vi "Alarm-102.vi"() -> ()   [LabVIEW 2009]
panel:
  out "³Ñ¤UªººÎ¯v®É¶¡":string
  in  "MINUTE":i32
  in  "HOUR":i32
  in  "stop":bool
  out "TIME":T1
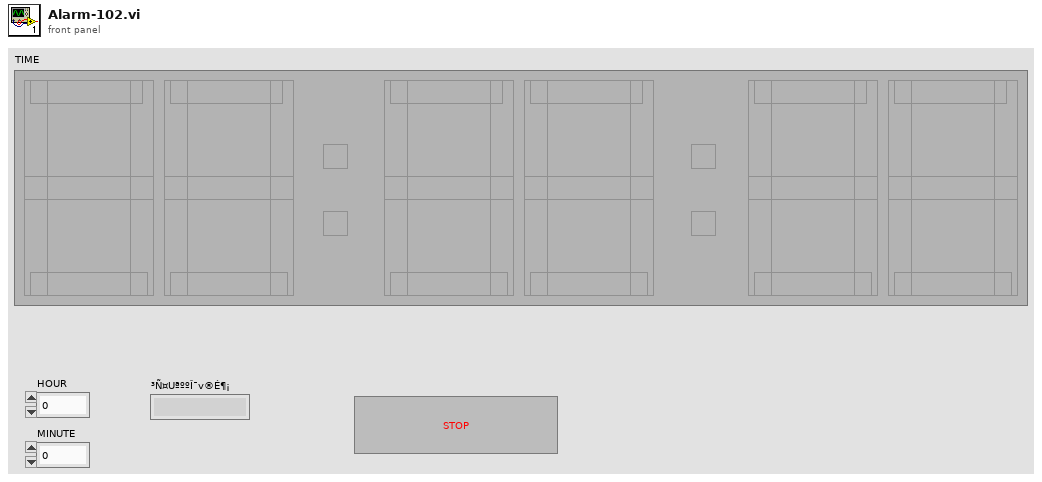
[diagram p1: front panel]
types:
  T1 = cluster{"Cluster":cluster{"Boolean 6":bool, "Boolean":bool, "Boolean 2":bool, "Boolean 7":bool, "Boolean 3":bool, "Boolean 4":bool, "Boolean 5":bool}, "Cluster 2":cluster{"Boolean 6":bool, "Boolean":bool, "Boolean 2":bool, "Boolean 7":bool, "Boolean 3":bool, "Boolean 4":bool, "Boolean 5":bool}, "Cluster 3":cluster{"Boolean 6":bool, "Boolean":bool, "Boolean 2":bool, "Boolean 7":bool, "Boolean 3":bool, "Boolean 4":bool, "Boolean 5":bool}, "Cluster 4":cluster{"Boolean 6":bool, "Boolean":bool, "Boolean 2":bool, "Boolean 7":bool, "Boolean 3":bool, "Boolean 4":bool, "Boolean 5":bool}, "Cluster 5":cluster{"Boolean 6":bool, "Boolean":bool, "Boolean 2":bool, "Boolean 7":bool, "Boolean 3":bool, "Boolean 4":bool, "Boolean 5":bool}, "Cluster 6":cluster{"Boolean 6":bool, "Boolean":bool, "Boolean 2":bool, "Boolean 7":bool, "Boolean 3":bool, "Boolean 4":bool, "Boolean 5":bool}, "sec1":bool, "sec2":bool, "sec2 2":bool, "sec1 2":bool}
  T2 = cluster{"Boolean 6":bool, "Boolean":bool, "Boolean 2":bool, "Boolean 7":bool, "Boolean 3":bool, "Boolean 4":bool, "Boolean 5":bool}[]
  T3 = typedef "LVDateTimeRec.ctl" = cluster{"fractional second":dbl, "second":i32, "minute":i32, "hour":i32, "day of month":i32, "month":i32, "year":i32, "day of week":i32, "day of year":i32, "DST":i32}
  T4 = cluster{"Boolean 6":bool, "Boolean":bool, "Boolean 2":bool, "Boolean 7":bool, "Boolean 3":bool, "Boolean 4":bool, "Boolean 5":bool}
  T5 = cluster{"second":i32, "minute":i32, "hour":i32, "day of month":i32, "month":i32, "year":i32, "day of week":i32, "day of year":i32, "is DST":i32}
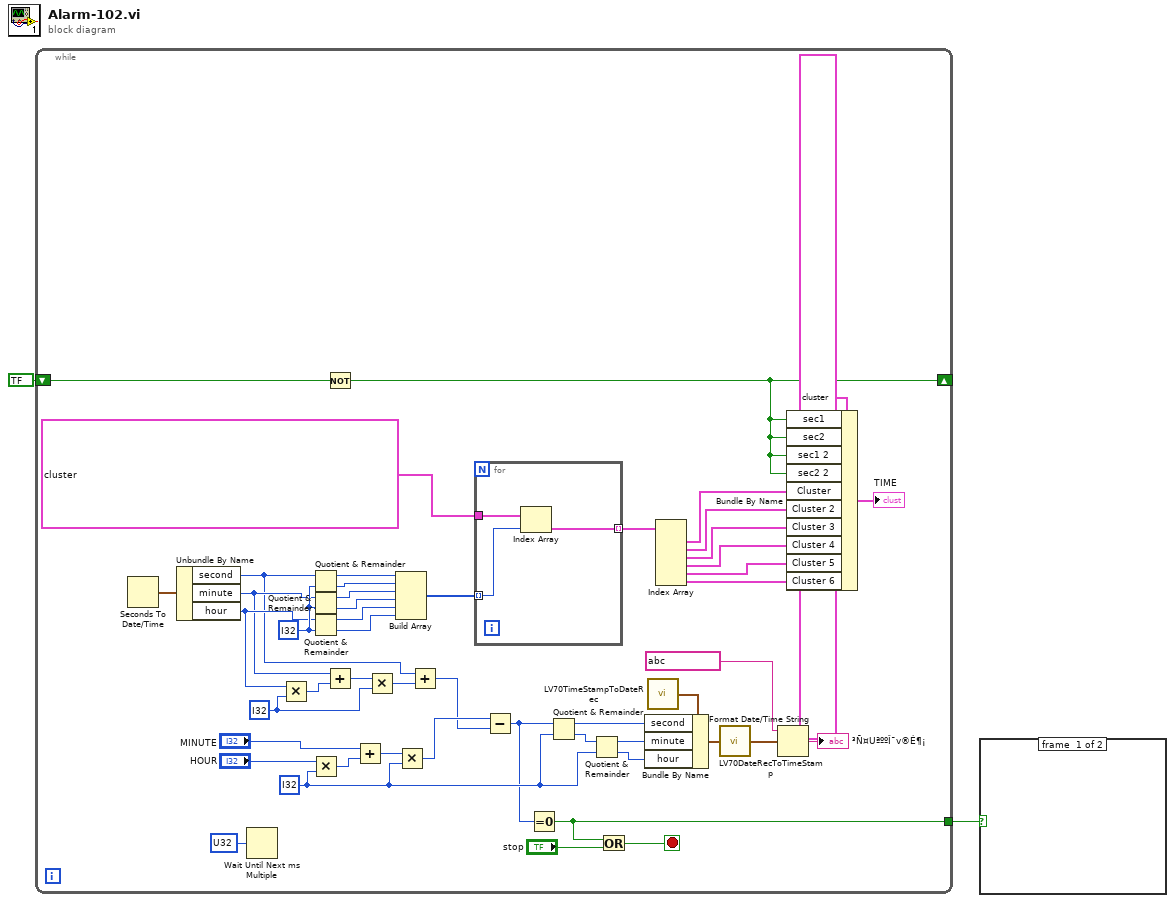
[diagram p0: block diagram]
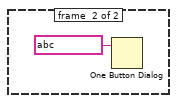
[diagram p2: hidden frame]
diagram:
  n1 = while {
    shift-right: [w30] -> _
    shift-left: bool ? -> [w31]
    tunnel: [w5] -> w1
    stop <- w3 stop-if-true
    w15 = i32 ? ("y")
    w25 = i32 ? ("y")
    w50 = i32 ? ("y")
    n2 = Seconds To Date/Time() -> (date time rec=w51:T3)  [unwired: 2 in]
    n3 = Unbundle By Name(w51) -> ("second"=w23:i32, "minute"=w27:i32, "hour"=w29:i32)
    n4 = Wait Until Next ms Multiple(millisecond multiple=u32 ?) -> ()  [unwired: 1 out]
    n5 = Multiply(x=w29, y=w25) -> (x*y=w28:i32)
    n6 = Quotient & Remainder(x=w23, y=w50) -> (x-y*floor(x/y)=w49:i32, floor(x/y)=w48:i32)
    n7 = Quotient & Remainder(x=w27, y=w50) -> (x-y*floor(x/y)=w47:i32, floor(x/y)=w46:i32)
    n8 = Quotient & Remainder(x=w29, y=w50) -> (x-y*floor(x/y)=w45:i32, floor(x/y)=w44:i32)
    n9 = Multiply(x="HOUR", y=w15) -> (x*y=w21:i32)
    n10 = Not(x=w31) -> (.not. x?=w30:bool)
    n11 = Add(x=w27, y=w28) -> (x+y=w26:i32)
    n12 = Add(x="MINUTE", y=w21) -> (x+y=w22:i32)
    n13 = Multiply(x=w26, y=w25) -> (x*y=w24:i32)
    n14 = Build Array(w49, w48, w47, w46, w45, w44) -> (w43:i32[])
    n15 = Multiply(x=w22, y=w15) -> (x*y=w18:i32)
    n16 = Add(x=w23, y=w24) -> (x+y=w17:i32)
    n17 = for {
      tunnel: w43 -> [w53] mode=indexing
      tunnel: T2 ? -> [w54]
      tunnel: [w52] -> w40 mode=indexing
      n18 = Index Array(array=w54, index=w53) -> (element=w52:T4)
    }
    n19 = Subtract(x=w18, y=w17) -> (x-y=w6:i32)
    n20 = Equal To 0?(x=w6) -> (x = 0?=w5:bool)
    n21 = Quotient & Remainder(x=w6, y=w15) -> (x-y*floor(x/y)=w11:i32, floor(x/y)=w16:i32)
    n22 = Quotient & Remainder(x=w16, y=w15) -> (x-y*floor(x/y)=w9:i32, floor(x/y)=w8:i32)
    n23 = Or(x=w5, y="stop") -> (x .or. y?=w3:bool)
    n24 = call <vilib>:"LV70TimeStampToDateRec.vi"() -> ("date time rec"=w14:T5)  [unwired: 1 in]
    n25 = Bundle By Name(cluster=w14, "second"=w11, "minute"=w9, "hour"=w8) -> (w13:T5)
    n26 = Index Array(array=w40) -> (element #1=w39:T4, element #2=w38:T4, element #3=w37:T4, element #4=w36:T4, element #5=w35:T4, element #6=w34:T4)  [unwired: 6 in]
    n27 = call <vilib>:"LV70DateRecToTimeStamp.vi"("date time rec"=w13) -> ("Time Stamp"=w10:timestamp)
    n28 = Format Date/Time String(time format string (%c)=string ?, seconds (now)=w10) -> (date/time string=→"³Ñ¤UªººÎ¯v®É¶¡":string)  [unwired: 1 in]
    n29 = Bundle By Name(cluster=T1 ? ("Cluster 2"), "sec1"=w30, "sec2"=w30, "sec1 2"=w30, "sec2 2"=w30, "Cluster"=w39, "Cluster 2"=w38, "Cluster 3"=w37, "Cluster 4"=w36, "Cluster 5"=w35, "Cluster 6"=w34) -> (→"TIME":T1)
  }
  n30 = case shown="True" w1 {
    frame #0 {
    }
    frame #1 {
      n31 = One Button Dialog(message=string ?) -> ()  [unwired: 1 in, 1 out]
    }
  }
